vi "SMT_Query Cell Transfer.vi"(0 "Traceability 引用句柄":refnum<k24>, 1 "OriginalEquipID":string, 2 "ComputerName":string, 3 "tblName":string, 5 "LoadID":string, 7 "StartDate":string, 9 "EndDate":string, 11 "error in (no error)":errorcluster caption="错误输入（无错误）", 12 "DestinationEquipID":string, 13 "Type":string) -> (4 "Traceability 引用句柄输出":refnum<k24>, 6 ".NET:System.Data.DataSet":T1={"CaseSensitive"=FALSE, "Container"=refnum, "DataSetName"="", "DefaultViewManager"=refnum, "DesignMode"=FALSE, "EnforceConstraints"=FALSE, "ExtendedProperties"=refnum, "HasErrors"=FALSE, "IsInitialized"=FALSE, "Locale"=refnum, "Namespace"="", "Prefix"="", "Relations"=refnum, "RemotingFormat"=0, "SchemaSerializationMode"=1, "Site"=refnum, "Tables"=refnum} {"SchemaSerializationMode" items=["IncludeSchema"=1, "ExcludeSchema"=2]; "RemotingFormat" items=["Xml", "Binary"]}, 15 "error out":errorcluster caption="错误输出")   [LabVIEW 2014, in "Traceability.lvlib"]
uses:
  D:/webservice/Traceability.dll
  Traceability.dll
  System.Data
  Traceability.lvlib
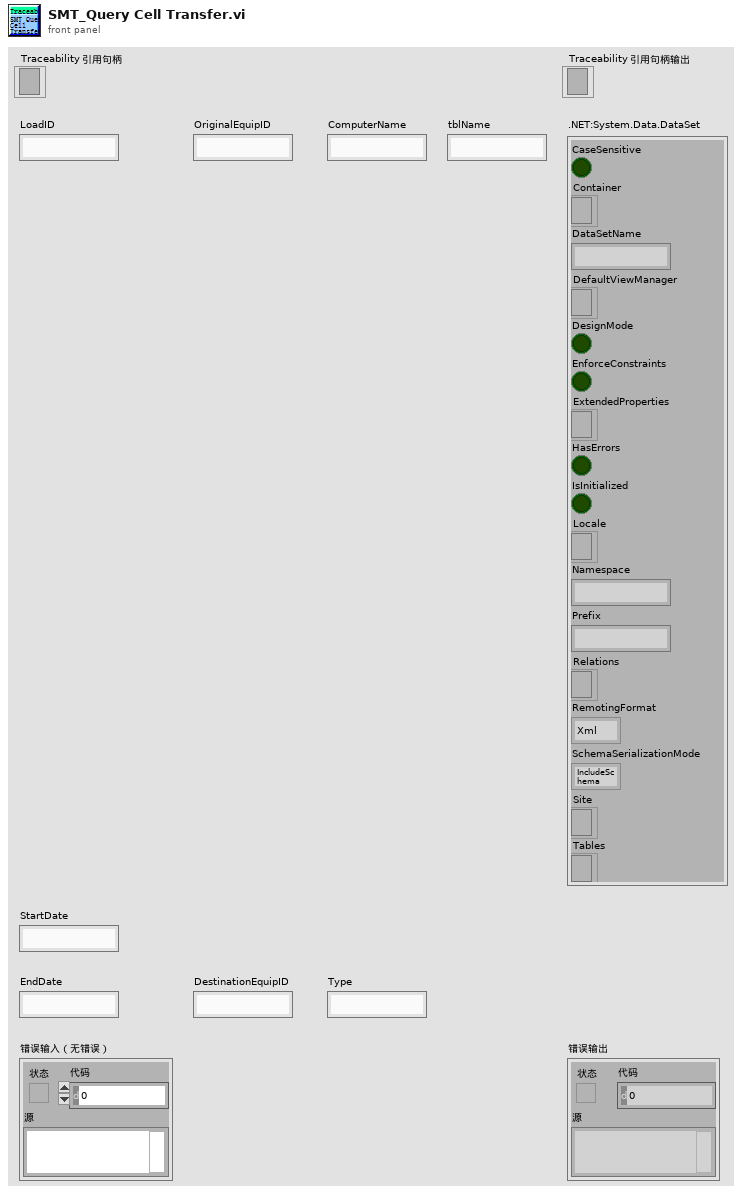
[diagram p1: front panel]
types:
  T1 = cluster{"CaseSensitive":bool, "Container":refnum<k24>, "DataSetName":string, "DefaultViewManager":refnum<k24>, "DesignMode":bool, "EnforceConstraints":bool, "ExtendedProperties":refnum<k24>, "HasErrors":bool, "IsInitialized":bool, "Locale":refnum<k24>, "Namespace":string, "Prefix":string, "Relations":refnum<k24>, "RemotingFormat":i32, "SchemaSerializationMode":i32, "Site":refnum<k24>, "Tables":refnum<k24>}
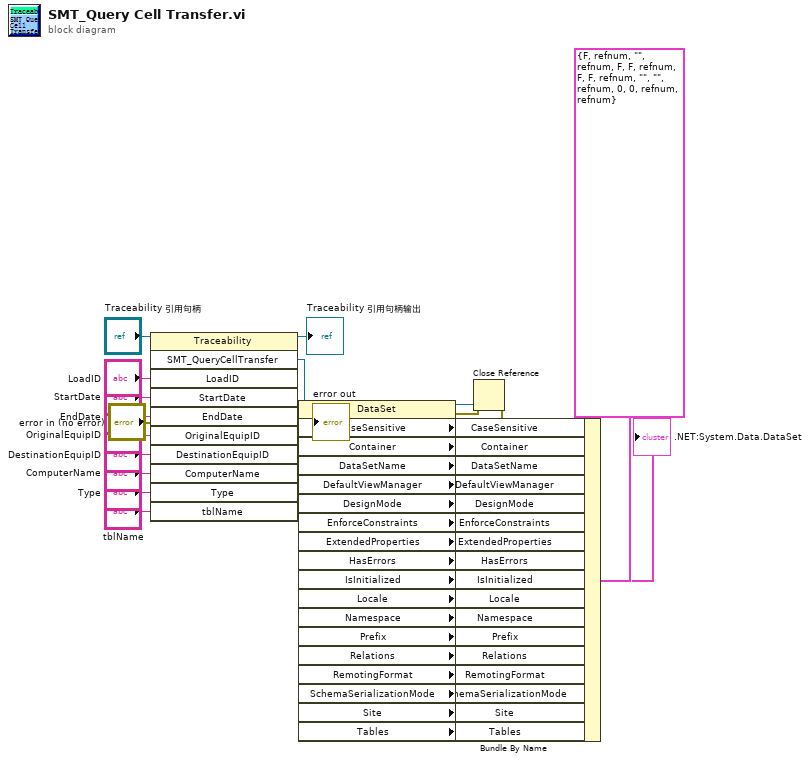
[diagram p0: block diagram]
diagram:
  n1 = invoke class="Traceability" method="SMT_QueryCellTransfer"(reference="Traceability 引用句柄", error in="error in (no error)", "LoadID"="LoadID", "StartDate"="StartDate", "EndDate"="EndDate", "OriginalEquipID"="OriginalEquipID", "DestinationEquipID"="DestinationEquipID", "ComputerName"="ComputerName", "Type"="Type", "tblName"="tblName") -> (reference out=→"Traceability 引用句柄输出":refnum<k24>, error out=w4:errorcluster, "SMT_QueryCellTransfer"=w32:refnum<k24>)  [unwired: 1 in, 8 out]
  n2 = property class="DataSet"(reference=w32, error in=w4) -> (reference out=w3:refnum<k24>, error out=w2:errorcluster, "CaseSensitive"=w29:bool, "Container"=w28:refnum<k24>, "DataSetName"=w27:string, "DefaultViewManager"=w26:refnum<k24>, "DesignMode"=w25:bool, "EnforceConstraints"=w24:bool, "ExtendedProperties"=w23:refnum<k24>, "HasErrors"=w22:bool, "IsInitialized"=w21:bool, "Locale"=w20:refnum<k24>, "Namespace"=w19:string, "Prefix"=w18:string, "Relations"=w17:refnum<k24>, "RemotingFormat"=w16:i32, "SchemaSerializationMode"=w15:i32, "Site"=w14:refnum<k24>, "Tables"=w13:refnum<k24>)
  n3 = Bundle By Name(cluster=T1 {"CaseSensitive"=FALSE, "Container"=refnum, "DataSetName"="", "DefaultViewManager"=refnum, "DesignMode"=FALSE, "EnforceConstraints"=FALSE, "ExtendedProperties"=refnum, "HasErrors"=FALSE, "IsInitialized"=FALSE, "Locale"=refnum, "Namespace"="", "Prefix"="", "Relations"=refnum, "RemotingFormat"=0, "SchemaSerializationMode"=0, "Site"=refnum, "Tables"=refnum} (".NET:System.Data.DataSet"), "CaseSensitive"=w29, "Container"=w28, "DataSetName"=w27, "DefaultViewManager"=w26, "DesignMode"=w25, "EnforceConstraints"=w24, "ExtendedProperties"=w23, "HasErrors"=w22, "IsInitialized"=w21, "Locale"=w20, "Namespace"=w19, "Prefix"=w18, "Relations"=w17, "RemotingFormat"=w16, "SchemaSerializationMode"=w15, "Site"=w14, "Tables"=w13) -> (→".NET:System.Data.DataSet":T1)
  n4 = Close Reference(reference=w3, error in (no error)=w2) -> (error out=→"error out":errorcluster)
